vi "Save_Destinations.vi"(8 "error in (no error)":errorcluster, 11 "AB_Deploy_EXE in":refnum<class "AB_Deploy_EXE.lvclass">) -> (0 "error out":errorcluster, 3 "AB_Deploy_EXE out":refnum<class "AB_Deploy_EXE.lvclass">)   [LabVIEW 2020, in "AB_Deploy_EXE.lvclass"]
uses:
  <vilib>/AppBuilder/AB_Classes/DeployableEXE/AB_Deploy_EXE.lvclass
  <vilib>/AppBuilder/AB_Classes/DeployableEXE/AB_Deploy_EXE.lvclass/AB_Deploy_EXE.ctl
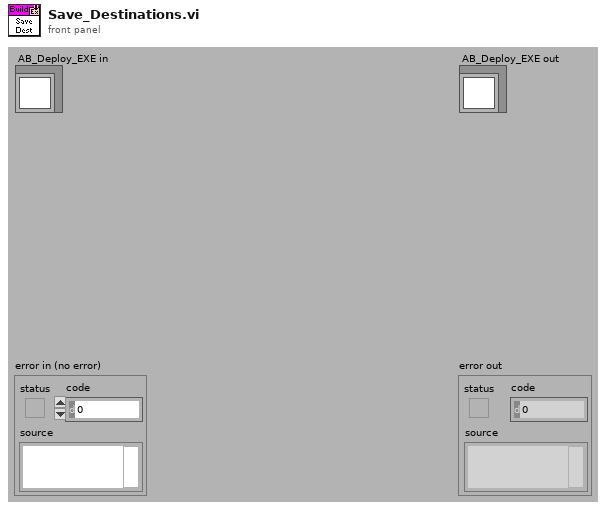
[diagram p1: front panel]
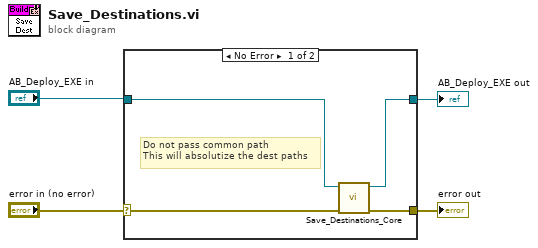
[diagram p0: block diagram]
diagram:
  n1 = case shown="No Error" "error in (no error)" {
    selector: "error in (no error)" -> [w5 w9]
    tunnel: [w8 w9] -> w2
    tunnel: "AB_Deploy_EXE in" -> [w7 w10]
    tunnel: [w6 w10] -> w3
    frame No Error {
      # "Do not pass common path\nThis will absolutize the dest paths"
      n2 = call-dynamic "Save_Destinations_Core.vi"("error in (no error)"=w5, "AB_Build in"=w7) -> ("error out"=w8:errorcluster, "AB_Build out"=w6:refnum<class "AB_Deploy_EXE.lvclass">)  [unwired: 8 in]
    }
    frame Error {
    }
  }
  "error out" <- w2
  "AB_Deploy_EXE out" <- w3
